vi "Cont Measure Voltage.vi"() -> ()   [LabVIEW 2012]
uses:
  <vilib>/DAQmx/create/channels.llb/DAQmx Create Channel (AI-Voltage-Basic).vi
  <vilib>/DAQmx/configure/timing.llb/DAQmx Timing (Sample Clock).vi
  <vilib>/DAQmx/read.llb/DAQmx Read (Analog 2D DBL NChan NSamp).vi
panel:
  in  "stop":bool
  in  "rate":dbl=1000.0 format="%0.2f"
  out "data":dbl[][](graph)
  in  "physical channels":tag
  out "error out":errorcluster
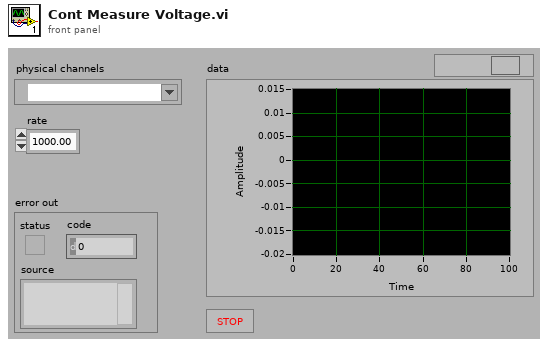
[diagram p1: front panel]
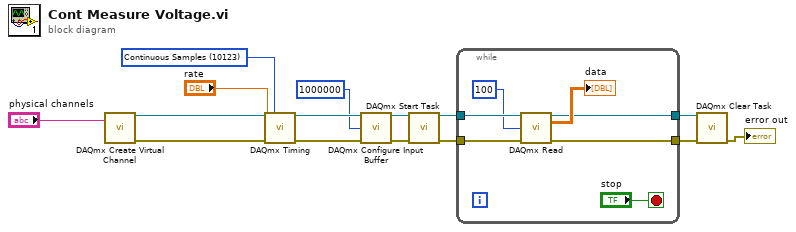
[diagram p0: block diagram]
diagram:
  w5 = 10123 items=["Finite Samples"=10178, "Continuous Samples"=10123, "Hardware Timed Single Point"=12522] ("sample mode")
  n1 = call-poly <vilib>:"DAQmx Create Virtual Channel.vi"("physical channels"="physical channels") -> ("task out"=w7:refnum<k21>, "error out"=w8:errorcluster)  [unwired: 13 in]
  n2 = call-poly <vilib>:"DAQmx Timing.vi"("task/channels in"=w7, "sample mode"=w5, "rate"="rate", "error in"=w8) -> ("task out"=w12:refnum<k21>, "error out"=w14:errorcluster)  [unwired: 10 in]
  n3 = call <vilib>:"DAQmx Configure Input Buffer.vi"("task/channels in"=w12, "buffer size (in samples per channel)"=u32 1000000, "error in"=w14) -> ("task out"=w13:refnum<k21>, "error out"=w15:errorcluster)  [unwired: 11 in]
  n4 = call <vilib>:"DAQmx Start Task.vi"("task/channels in"=w13, "error in"=w15) -> ("task out"=w10:refnum<k21>, "error out"=w11:errorcluster)  [unwired: 12 in]
  n5 = while {
    tunnel: w11 -> [w22]
    tunnel: w10 -> [w21]
    tunnel: [w18] -> w3
    tunnel: [w17] -> w2
    stop <- "stop" stop-if-true
    n6 = call-poly <vilib>:"DAQmx Read.vi"("task/channels in"=w21, "number of samples per channel"=100, "error in"=w22) -> ("task out"=w18:refnum<k21>, "data"=→"data":dbl[][], "error out"=w17:errorcluster)  [unwired: 10 in]
  }
  n7 = call <vilib>:"DAQmx Clear Task.vi"("task in"=w3, "error in"=w2) -> ("error out"=→"error out":errorcluster)  [unwired: 13 in]
